vi "VIHasSubVIInAProjectLibrary.vi"() -> (0 "error out":errorcluster, 3 "Waveform Graph":waveform(dbl)(graph))   [LabVIEW 2012]
uses:
  <vilib>/measure/mascope.llb/Amplitude and Levels 1 chan.vi
  <vilib>/measure/mamon.llb/Waveform Peak Detection for 1 Chan.vi
  <vilib>/measure/NI_MABase.lvlib
  <vilib>/measure/NI_MAPro.lvlib
panel:
  out "Locations":dbl[](array[numeric]) format="%.2p"
  out "amplitude":dbl format="%.2p"
  out "2nd Derivatives":dbl[](array[numeric]) format="%.2p"
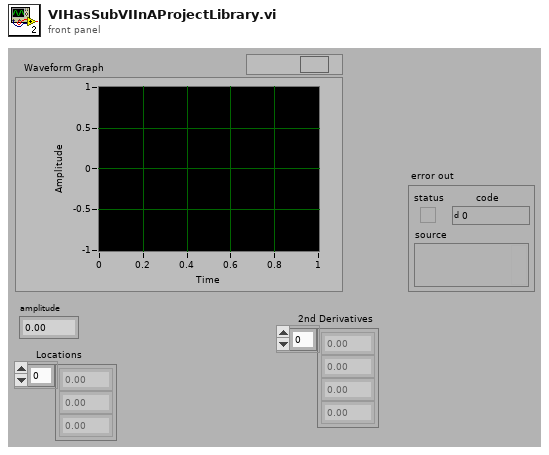
[diagram p1: front panel]
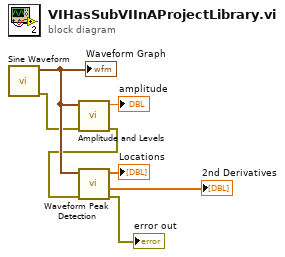
[diagram p0: block diagram]
diagram:
  n1 = call <vilib>:"Sine Waveform.vi"() -> ("error out"=w3:errorcluster, "signal out"=w7:waveform(dbl))  [unwired: 7 in, 3 out]
  "Waveform Graph" <- w7
  n2 = call-poly <vilib>:"Amplitude and Levels.vi"("error in (no error)"=w3, "signal in"=w7) -> ("error out"=w2:errorcluster, "amplitude"=→"amplitude":dbl)  [unwired: 1 in, 7 out]
  n3 = call-poly <vilib>:"Waveform Peak Detection.vi"("error in"=w2, "Signal In"=w7) -> ("error out"=→"error out":errorcluster, "2nd Derivatives"=→"2nd Derivatives":dbl[], "Locations"=→"Locations":dbl[])  [unwired: 5 in, 2 out]
